vi "CallBack Tag.vi"(6 "Variant":variant, 8 "error in (no error)":errorcluster, 9 "Old Values":string[][](array[string]), 10 "object ref in":T1, 11 "Table Change":T2) -> (0 "error out":errorcluster)   [LabVIEW 2014, in "control module editor.lvclass"]
uses:
  control module editor.lvclass
  Table API/Table Manager/Cell Change.ctl
  Table API/Table Manager/object ref.ctl
  Configuration Editor/Classes/Engine Parent/Engine Parent Editor Node.lvclass
  Configuration Editor/Classes/Module editor node/module editor node.lvclass
  <vilib>/NI/Tag Bus Module Framework/channel/TBM channel.lvclass
  configuration/control module configuration.lvclass
  configuration/control module configuration.lvclass/control module configuration.ctl
  <vilib>/NI/Tag Bus/tag/tag descriptor.lvclass/tag descriptor.ctl
  <vilib>/NI/Tag Bus/tag/read tag name.vi
  <vilib>/NI/Tag Bus/tag/tag descriptor.lvclass
  Table API/Table Manager.lvlib
  Table API/Table Manager/Table Manager.lvclass
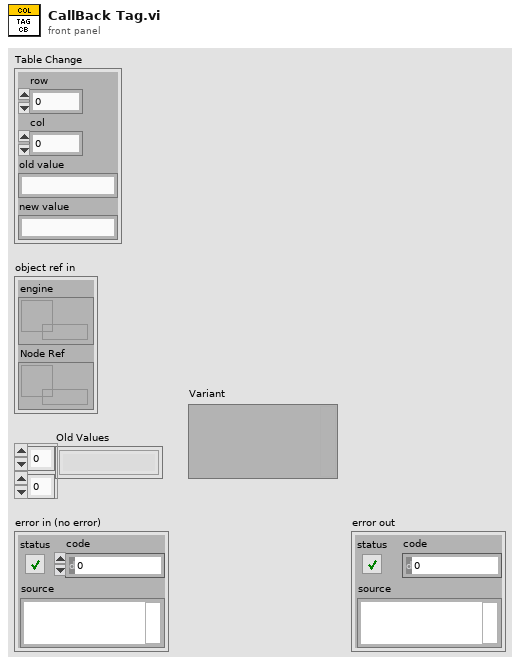
[diagram p1: front panel]
types:
  T1 = typedef "Table Manager.lvlib/Table Manager.lvclass/object ref.ctl" = cluster{"engine":refnum<data-value>, "Node Ref":refnum<data-value>}
  T2 = typedef "Table Manager.lvlib/Cell Change.ctl" = cluster{"row":i32, "col":i32, "old value":string, "new value":string}
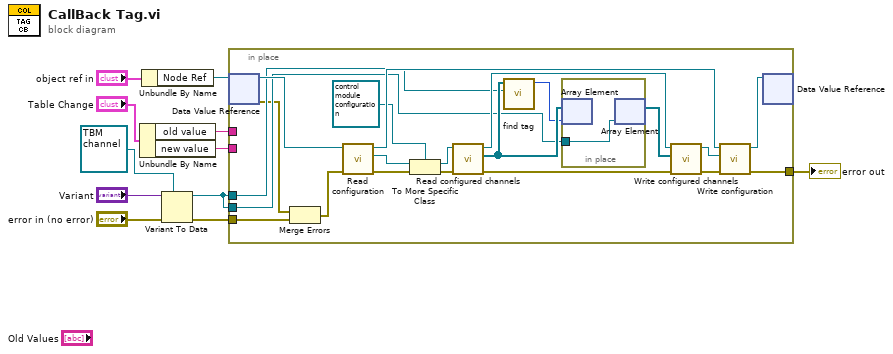
[diagram p0: block diagram]
diagram:
  n1 = Unbundle By Name("Table Change") -> ("old value"=w10:string, "new value"=w9:string)
  n2 = Unbundle By Name("object ref in") -> ("Node Ref"=w11:refnum<data-value>)
  n3 = Variant To Data(error in="error in (no error)", type=refnum<class "TBM channel.lvclass"> refnum ("channel"), Variant="Variant") -> (data=w3:refnum<class "TBM channel.lvclass">, error out=w1:errorcluster)
  n4 = in-place {
    in-place-border: [w21] -> w8
    in-place-border: w10 -> [_]
    in-place-border: w9 -> [_]
    in-place-border: w3 -> [w17]
    in-place-border: w3 -> [w15]
    in-place-border: w1 -> [w14]
    n5 = in-place-dvr #1(w11) -> (w30:refnum<class "module editor node.lvclass">, w13:errorcluster)
    n6 = Merge Errors(w13, w14) -> (w12:errorcluster)
    n7 = call-dynamic "Read configuration.vi"("error in"=w12, "NISE_CEF_serializable node in"=w30) -> ("error out"=w25:errorcluster, "configuration"=w27:refnum<class "NISE_CEF_serializable configuration.lvclass">, "NISE_CEF_serializable node out"=w31:refnum<class "module editor node.lvclass">)  [unwired: 7 in]
    n8 = To More Specific Class(target class=refnum<class "control module configuration.lvclass"> refnum ("fixed channel configuration"), reference=w27, error in=w25) -> (specific class reference=w28:refnum<class "control module configuration.lvclass">, error out=w24:errorcluster)
    n9 = call "Read configured channels.vi"("error in (no error)"=w24, "control module configuration in"=w28) -> ("error out"=w23:errorcluster, "configured channels"=w18:refnum<class "TBM channel.lvclass">[], "control module configuration out"=w20:refnum<class "control module configuration.lvclass">)  [unwired: 7 in]
    n10 = call <vilib>:"find tag.vi"("tag"=w17, "tags in"=w18) -> ("index"=w16:i32)  [unwired: 9 in]
    n11 = in-place {
      in-place-border: w15 -> [w33]
      n12 = in-place-array #2(w18, w16) -> ()  [unwired: 1 out]
      n13 = in-place-array #2(w33) -> (w19:refnum<class "TBM channel.lvclass">[])  [unwired: 1 out]
    }
    n14 = call "Write configured channels.vi"("error in (no error)"=w23, "configured channels"=w19, "control module configuration in"=w20) -> ("error out"=w22:errorcluster, "control module configuration out"=w26:refnum<class "control module configuration.lvclass">)  [unwired: 7 in]
    n15 = call-dynamic "Write configuration.vi"("error in"=w22, "configuration"=w26, "NISE_CEF_serializable node in"=w31) -> ("error out"=w21:errorcluster, "NISE_CEF_serializable node out"=w32:refnum<class "module editor node.lvclass">)  [unwired: 7 in]
    n16 = in-place-dvr #1(w32) -> ()  [unwired: 2 out]
  }
  "error out" <- w8
